vi "Read database.vi"(0 "database":string="database1.mdb", 1 "显示项":string[](array[string])=["top 100 *"], 5 "组合框":string(combo)="CODMn", 9 "condition":string="where 时间 between #2020/03/27 14:26:18 # and #2020/04/26 14:26:18# order by 时间 desc", 11 "error in (no error)":errorcluster caption="错误输入（无错误）") -> (3 "columns":string[](array[string]), 4 "表格":string[][](table), 6 "column information":T2(array[cluster]), 8 "foretime":string, 10 "lasttime":string, 15 "error out":errorcluster caption="错误输出")   [LabVIEW 2016]
uses:
  <vilib>/addons/database/Auxilliary.llb/DB Tools DataTypes.ctl
  <vilib>/Utility/sysdir.llb/System Directory Type.ctl
  <vilib>/addons/database/Connection.llb/DB Tools Open Connec (String).vi
  <vilib>/addons/database/_DB Variant To Data/Database Variant To Data.xnode
  <vilib>/addons/database/NI_Database_API.lvlib
panel:
  in  "精度(6)":i16=2
  out "data":variant[][](array[variant])
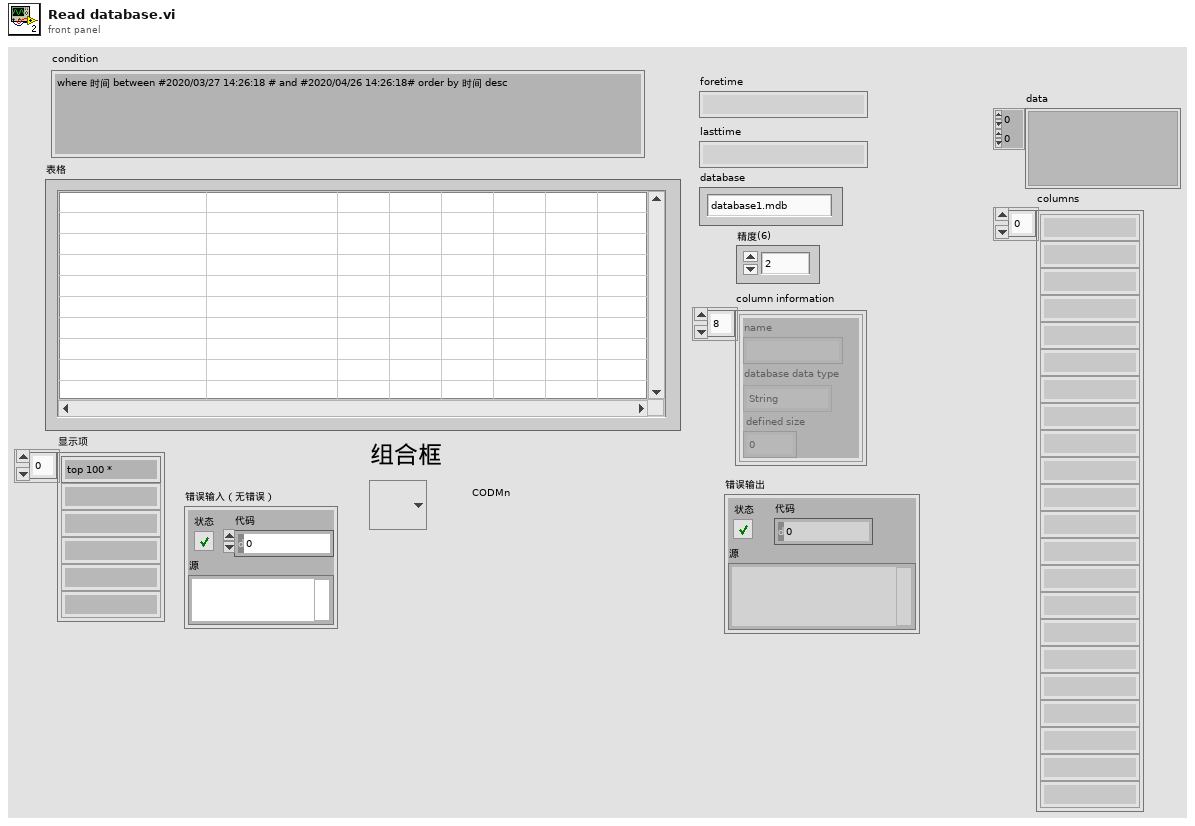
[diagram p1: front panel]
types:
  T1 = typedef "NI_Database_API.lvlib/DB Tools DataTypes.ctl" = enum16{"String", "Long (I32)", "Single (SGL)", "Double (DBL)", "Date/Time", "Binary"}
  T2 = cluster{"name":string, "database data type":T1, "defined size":i32}[]
  T3 = typedef "System Directory Type.ctl" = i32
  T4 = typedef "NI_Database_API.lvlib/Conn ObjectReference.ctl" = refnum<k1>
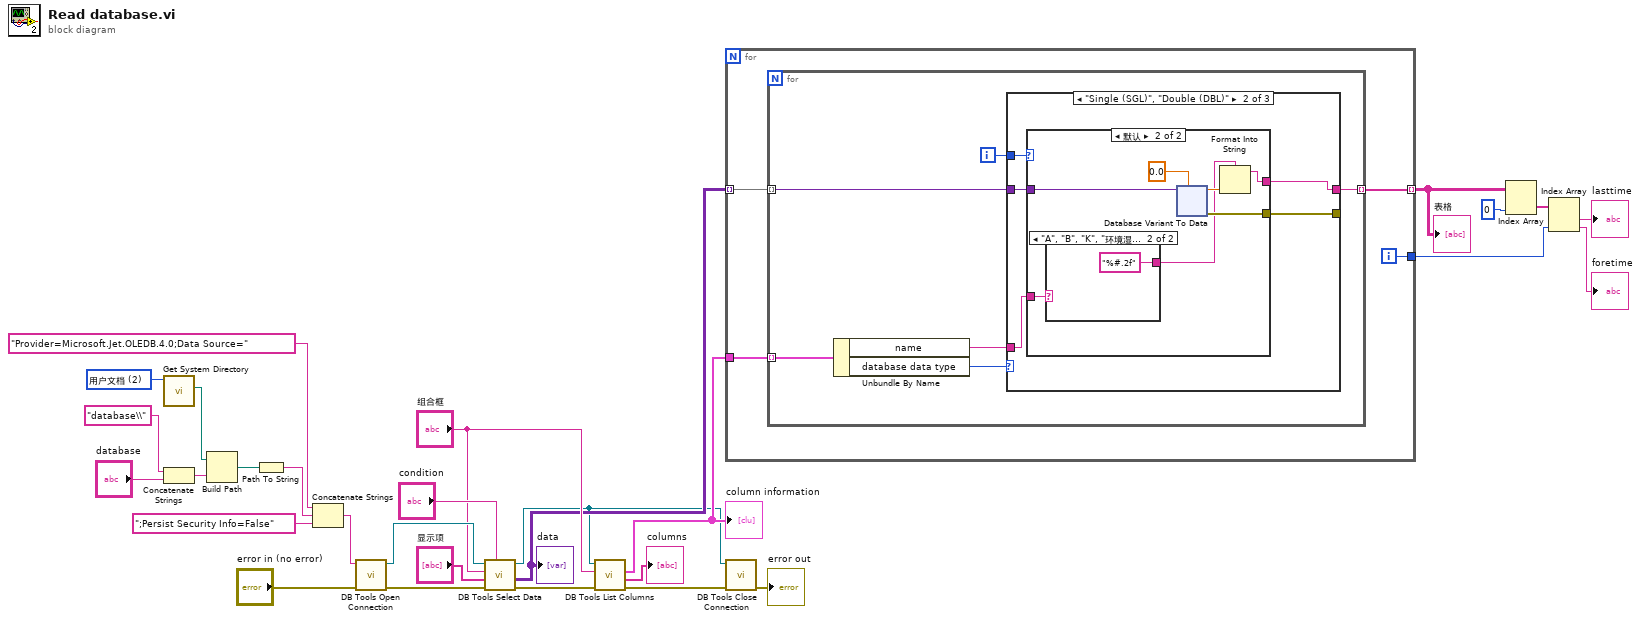
[diagram p0: block diagram]
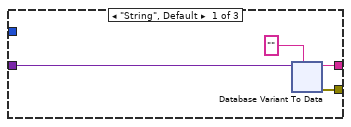
[diagram p2: hidden frame]
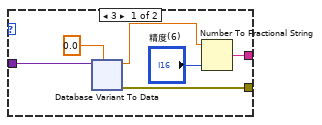
[diagram p3: hidden frame]
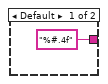
[diagram p4: hidden frame]
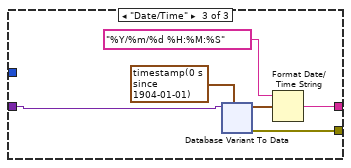
[diagram p5: hidden frame]
diagram:
  w16 = T3 2 items=["用户目录"=0, "用户桌面"=1, "用户文档"=2, "用户应用程序数据"=3, "用户设置"=4, "用户临时目录"=5, "公共文档"=6, "公共应用程序数据"=7, "公共设置"=8, "公共缓存"=13, "系统核心库"=9, "系统安装库"=10, "应用程序文件"=11, "启动盘根目录"=12] ("system directory type")
  n1 = call <vilib>:"Get System Directory.vi"("system directory type"=w16) -> ("system directory"=w15:path)  [unwired: 10 in]
  n2 = Concatenate Strings("database\\" ("名称或相对路径"), "database") -> (w12:string)
  n3 = Build Path(base path=w15, name or relative path=w12) -> (appended path=w17:path)
  n4 = Path To String(path=w17) -> (string=w18:string)
  n5 = Concatenate Strings("Provider=Microsoft.Jet.OLEDB.4.0;Data Source=", w18, ";Persist Security Info=False") -> (w14:string)
  n6 = call-poly <vilib>:"DB Tools Open Connection.vi"("error in (no error)"="error in (no error)", "connection information"=w14) -> ("error out"=w28:errorcluster, "connection reference"=w29:T4)  [unwired: 6 in]
  n7 = call <vilib>:"DB Tools Select Data.vi"("condition"="condition", "error in (no error)"=w28, "columns"="显示项", "table"="组合框", "connection reference"=w29) -> ("error out"=w27:errorcluster, "data"=w9:variant[][], "connection reference out"=w7:T4)  [unwired: 1 in]
  "data" <- w9
  n8 = call <vilib>:"DB Tools List Columns.vi"("error in (no error)"=w27, "table"="组合框", "connection reference"=w7) -> ("error out"=w21:errorcluster, "columns"=→"columns":string[], "column information"=w8:T2)  [unwired: 1 in, 1 out]
  "column information" <- w8
  n9 = for {
    tunnel: w9 -> [w33] mode=indexing
    tunnel: w8 -> [w32]
    tunnel: [w31] -> w5 mode=indexing
    tunnel: [w30] -> w1
    i -> [w30]
    n10 = for {
      tunnel: w33 -> [w38] mode=indexing
      tunnel: w32 -> [w37] mode=indexing
      tunnel: [w35] -> w31 mode=indexing
      i -> [w36]
      n11 = Unbundle By Name(w37) -> ("name"=w34:string, "database data type"=w39:T1)
      n12 = case shown="\"Single (SGL)\", \"Double (DBL)\"" w39 {
        tunnel: w38 -> [w43 w80 w165]
        tunnel: [w40 w79 w161] -> w35
        tunnel: w36 -> [_ w78 _]
        tunnel: [w41 w77 w160] -> _
        tunnel: w34 -> [_ w76 _]
        frame "String", Default {
          n13 = xnode "Database Variant To Data"("database variant"=w43, "type"="") -> ("data"=w40:string, "error out"=w41:errorcluster)  [unwired: 1 in]
        }
        frame "Single (SGL)", "Double (DBL)" {
          n14 = case shown="默认" w78 {
            tunnel: w80 -> [w86 w125]
            tunnel: [w84 w120] -> w79
            tunnel: [w81 w123] -> w77
            tunnel: w76 -> [_ w121]
            frame 3 {
              n15 = xnode "Database Variant To Data"("database variant"=w86, "type"=0.0) -> ("data"=w85:dbl, "error out"=w81:errorcluster)  [unwired: 1 in]
              n16 = Number To Fractional String(number=w85, precision (6)="精度(6)") -> (F-format string=w84:string)  [unwired: 2 in]
            }
            frame Default {
              n17 = case shown="\"A\", \"B\", \"K\", \"环境湿度\", \"环境温度\", \"加热实时温度\"" w121 {
                tunnel: ["%#.4f" ("格式字符串") "%#.2f" ("格式字符串")] -> w119
                frame Default {
                }
                frame "A", "B", "K", "环境湿度", "环境温度", "加热实时温度" {
                }
              }
              n18 = xnode "Database Variant To Data"("database variant"=w125, "type"=0.0) -> ("data"=w122:dbl, "error out"=w123:errorcluster)  [unwired: 1 in]
              n19 = Format Into String(format string=w119, w122) -> (resulting string=w120:string)  [unwired: 2 in, 1 out]
            }
          }
        }
        frame "Date/Time" {
          n20 = xnode "Database Variant To Data"("database variant"=w165, "type"=timestamp(0 s since 1904-01-01) ("当前时间")) -> ("data"=w164:timestamp, "error out"=w160:errorcluster)  [unwired: 1 in]
          n21 = Format Date/Time String(time format string (%c)="%Y/%m/%d %H:%M:%S" ("时间格式字符串(%c)"), seconds (now)=w164) -> (date/time string=w161:string)  [unwired: 1 in]
        }
      }
    }
  }
  "表格" <- w5
  n22 = call <vilib>:"DB Tools Close Connection.vi"("error in (no error)"=w21, "connection reference"=w7) -> ("error out"=→"error out":errorcluster)  [unwired: 5 in]
  n23 = Index Array(array=w5, index (col)=0 ("禁用的索引 (列)")) -> (element=w4:string[])  [unwired: 1 in]
  n24 = Index Array(array=w4, index #2=w1) -> (element #1=→"lasttime":string, element #2=→"foretime":string)  [unwired: 1 in]
